vi "LOG COUNT.vi"(8 "error in (no error)":errorcluster, 10 "LOG":bool, 11 "Binary counter in":refnum<class "Binary counter.lvclass">) -> (0 "error out":errorcluster, 3 "Binary counter out":refnum<class "Binary counter.lvclass">)   [LabVIEW 2020, in "Binary counter.lvlib" / "Binary counter.lvclass"]
uses:
  Binary counter.lvclass
  Binary counter.lvclass/Binary counter.ctl
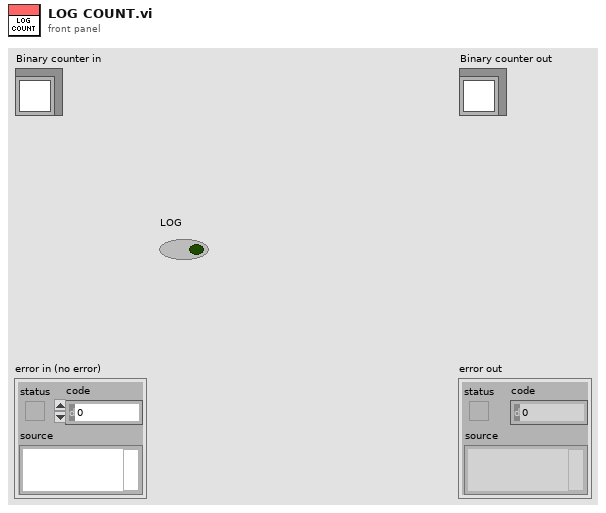
[diagram p1: front panel]
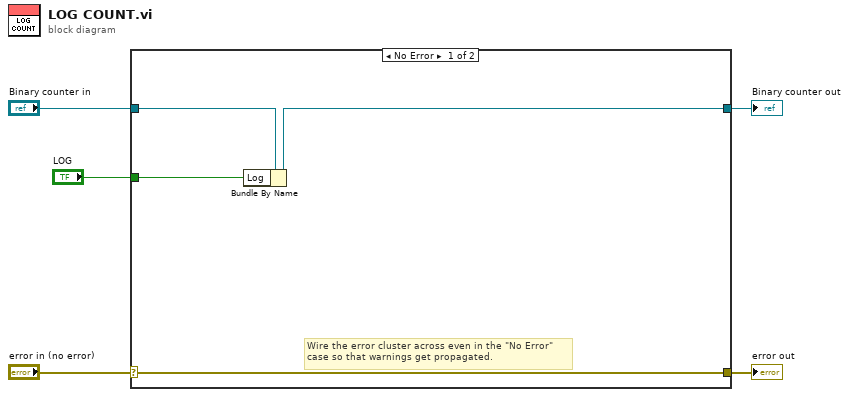
[diagram p0: block diagram]
diagram:
  n1 = case shown="No Error" "error in (no error)" {
    selector: "error in (no error)" -> [w9 w11]
    tunnel: [w9 w11] -> w4
    tunnel: [w7 w10] -> w2
    tunnel: "Binary counter in" -> [w8 w10]
    tunnel: "LOG" -> [w6 _]
    frame No Error {
      # "Wire the error cluster across even in the \"No Error\"\ncase so that warnings get propagated."
      n2 = Bundle By Name(cluster=w8, "Log"=w6) -> (w7:refnum<class "Binary counter.lvclass">)
    }
    frame Error {
    }
  }
  "error out" <- w4
  "Binary counter out" <- w2
